vi "Set_Parameter_Instrument (Json).vi"(8 "error in (no error)":errorcluster caption="entrée d'erreur (pas d'erreur)", 10 "Parameter (Json)":string, 11 "Flash_Jlink en entrée":refnum<class "Flash_Epox.lvclass">) -> (0 "error out":errorcluster caption="sortie d'erreur", 3 "Flash_Jlink en sortie":refnum<class "Flash_Epox.lvclass">)   [LabVIEW 2020, in "Library Test.lvlib" / "Flash_Epox.lvclass"]
uses:
  Flash_Epox.lvclass
  C:/Users/ngarcin/OneDrive - Altyor/Standard TB/Class/Test/Test (Default)/Test (Default).lvclass
  Commun VI/TypeDef/Commande Test/Commande Parameter Flash_eoxp.ctl
  Flash_Epox.lvclass/Flash_Epox.ctl
  JSON API/JSON Value/Set from JSON string.vi
  Test_Without_Instr/Test_Without_Inst.lvclass
  JSON API/JSON Value/JSON Value.lvclass
  JSON API/Variant JSON/Variant JSON.lvlib
  JSON API/Get Polymorphic/JSON GetSet.lvlib
  Commun VI/Library Commun.lvlib
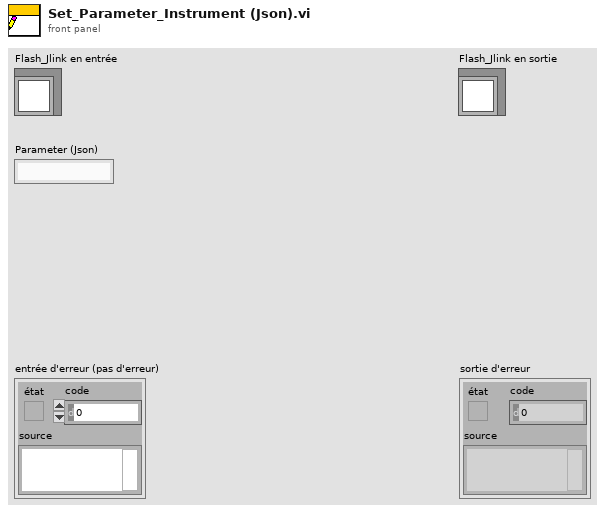
[diagram p1: front panel]
types:
  T1 = typedef "Library Commun.lvlib/Commande Parameter Flash_eoxp.ctl" = cluster{"Path FW ":path, "Working Directory":path, "Path Config":path}
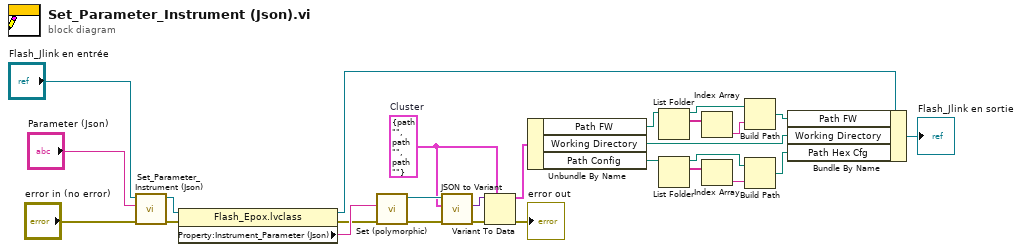
[diagram p0: block diagram]
diagram:
  w6 = T1 {"Path FW "=path "", "Working Directory"=path "", "Path Config"=path ""}  # Cluster
  n1 = call-parent "Set_Parameter_Instrument (Json).vi"("error in (no error)"="error in (no error)", "Parameter (Json)"="Parameter (Json)", "Test (Default) en entrée"="Flash_Jlink en entrée") -> ("error out"=w17:errorcluster, "Test (Default) en sortie"=w19:refnum<class "Flash_Epox.lvclass">)  [unwired: 7 in]
  n2 = property class="Flash_Epox.lvclass"(reference=w19, error in=w17) -> (reference out=w16:refnum<class "Flash_Epox.lvclass">, error out=w14:errorcluster, "Property:Instrument_Parameter (Json)"=w18:string)
  n3 = call-poly "Set (polymorphic).vi"("error in (no error)"=w14, "JSON stream"=w18) -> ("error out"=w21:errorcluster, "JSON Value out"=w23:refnum<class "JSON Value.lvclass">)  [unwired: 7 in, 1 out]
  n4 = call "JSON to Variant.vi"("error in (no error)"=w21, "Variant (Data Type)"=w6, "JSON Value"=w23) -> ("error out"=w22:errorcluster, "Variant out"=w20:variant)  [unwired: 7 in]
  n5 = Variant To Data(error in=w22, type=w6, Variant=w20) -> (data=w15:T1, error out=→"error out":errorcluster)
  n6 = Unbundle By Name(w15) -> ("Path FW"=w8:path, "Working Directory"=w12:path, "Path Config"=w3:path)
  n7 = List Folder(path=w8) -> (path out=w9:path, filenames=w11:string[])  [unwired: 3 in, 2 out]
  n8 = List Folder(path=w3) -> (path out=w5:path, filenames=w4:string[])  [unwired: 3 in, 2 out]
  n9 = Index Array(array=w11) -> (element=w10:string)  [unwired: 1 in]
  n10 = Index Array(array=w4) -> (element=w1:string)  [unwired: 1 in]
  n11 = Build Path(base path=w9, name or relative path=w10) -> (appended path=w7:path)
  n12 = Build Path(base path=w5, name or relative path=w1) -> (appended path=w2:path)
  n13 = Bundle By Name(cluster=w16, "Path FW"=w7, "Working Directory"=w12, "Path Hex Cfg"=w2) -> (→"Flash_Jlink en sortie":refnum<class "Flash_Epox.lvclass">)
